vi "GetTypeDefs.vi"(0 "ClassReaderNative in":refnum<class "ClassReaderNative.lvclass">, 5 "error in (no error)":errorcluster) -> (14 "ClassReaderNative out":refnum<class "ClassReaderNative.lvclass">, 15 "TypeDefs":T1[](array[typedef]), 19 "error out":errorcluster)   [LabVIEW 2012, in "ClassReaderNative.lvclass"]
uses:
  <resource>/Framework/Providers/Open_GDS/ClassProviders/Provider_LvNativeClass/ClassReaderNative_class/ClassReaderNative.lvclass
  <resource>/Framework/Providers/Open_GDS/UML/ReversedEngineering/ReversedEngineering TypeDefType.ctl
  <resource>/Framework/Providers/Open_GDS/UML/ReversedEngineering/ReversedEngineering AttributeInfoType.ctl
  <resource>/Framework/Providers/Open_GDS/ClassProviders/Common/CommonVIs/CommonVIs_AttributeDataType.ctl
  <resource>/Framework/Providers/Open_GDS/UML/UMLEditor/UMLEditor_VisibilityType.ctl
  <resource>/Framework/Providers/Open_GDS/ClassProviders/Provider_LvNativeClass/ClassReaderNative_class/ClassReaderNative.lvclass/ClassReaderNative.ctl
  <resource>/Framework/Providers/Open_GDS/ClassProviders/Provider_BaseClassInterface/ClassReader_class/ClassReader.lvclass
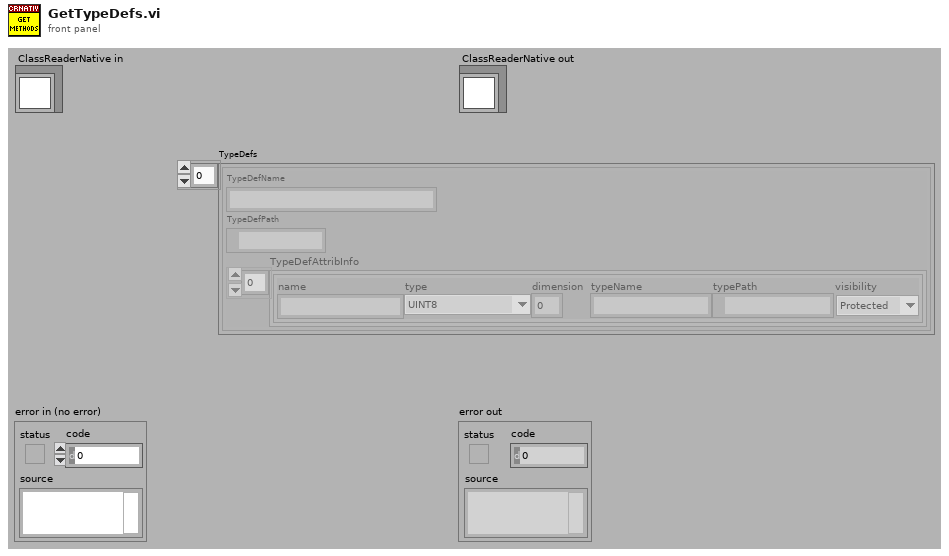
[diagram p1: front panel]
types:
  T1 = typedef "ReversedEngineering TypeDefType.ctl" = cluster{"TypeDefName":string, "TypeDefPath":path, "TypeDefAttribInfo":T2[]}
  T2 = typedef "ReversedEngineering AttributeInfoType.ctl" = cluster{"name":string, "type":T3, "dimension":i32, "typeName":string, "typePath":path, "visibility":T4}
  T3 = typedef "CommonVIs_AttributeDataType.ctl" = enum16{"UINT8", "INT8", "UINT16", "INT16", "UINT32", "INT32", "UINT64", "INT64", "SGL", "DBL", "EXT", "CSG", "CDB", "CXT", "TimeStamp", "STRING", "PATH", "BOOL", "ENUM", "RefNum", "VIRefNum", "LabVIEW Class", "Cluster", "Variant", "TypeDef", "Waveform", "LabVIEW Object", "Other"}
  T4 = typedef "UMLEditor_VisibilityType.ctl" = enum16{"Public", "Private", "Protected"}
  T5 = enum32{"invalid VI type", "Standard VI", "Control VI", "Global VI", "Polymorphic VI", "Configuration VI", "SubSystem", "Facade VI", "Method VI", "Statechart Diagram VI"}
  T6 = enum32{"not a control VI", "control", "typedef", "strict typedef"}
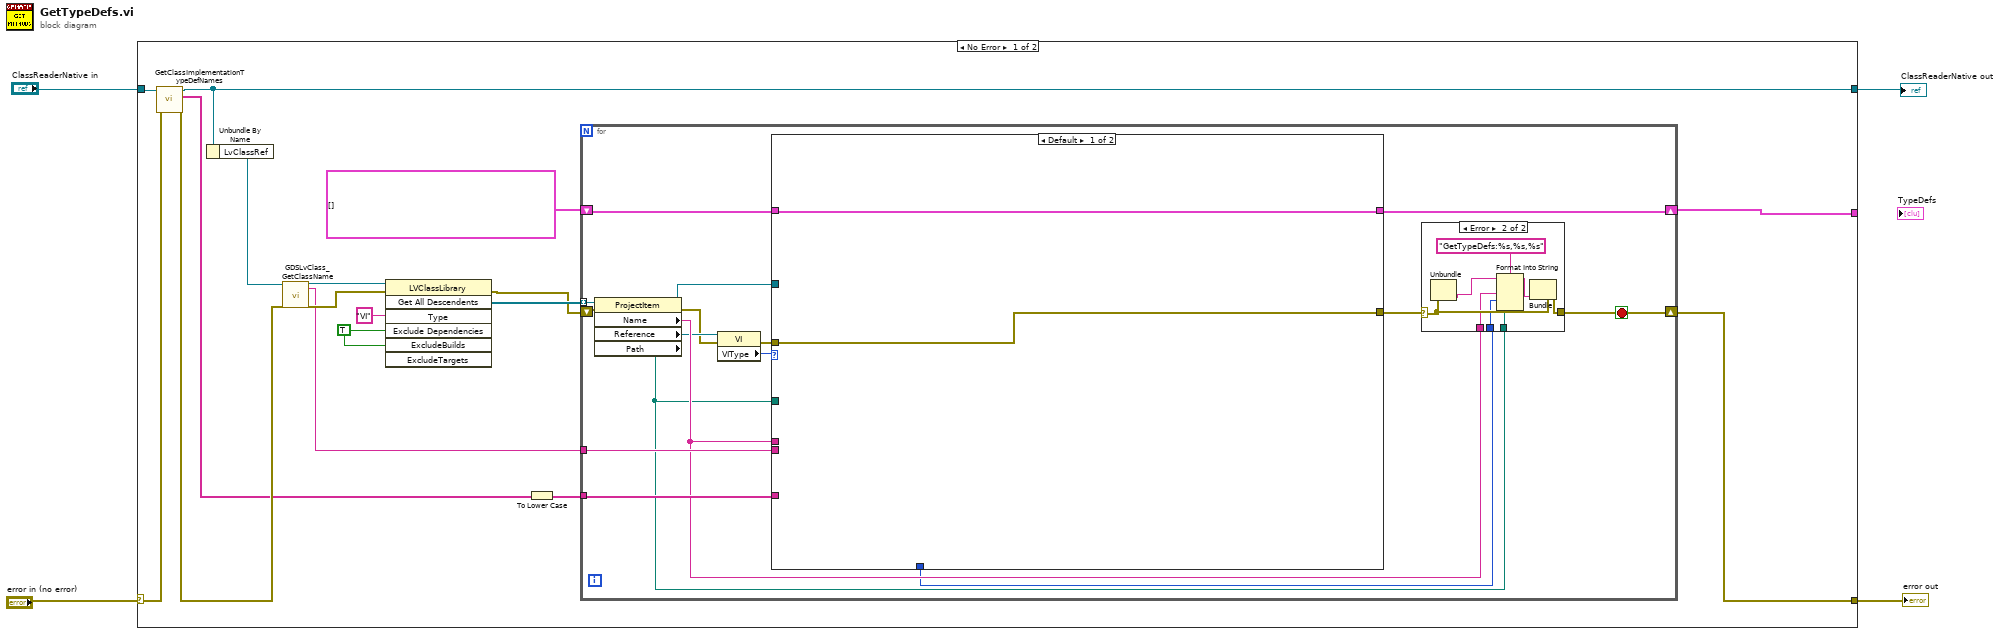
[diagram p0: block diagram]
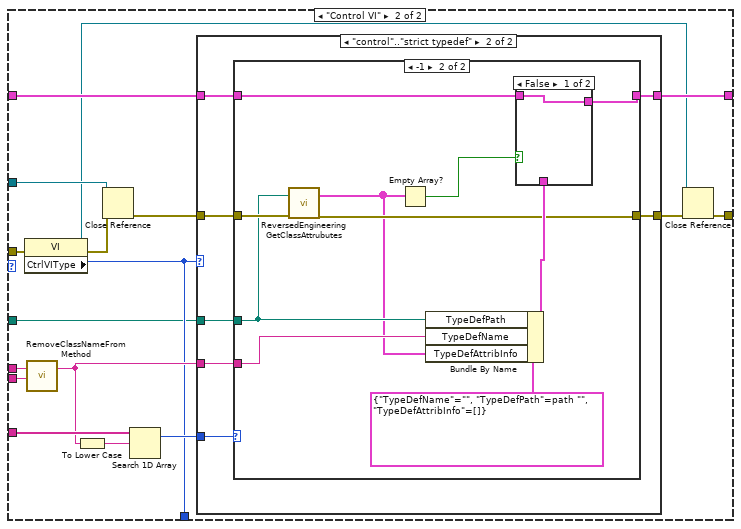
[diagram p2: hidden frame]
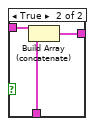
[diagram p5: hidden frame]
diagram:
  n1 = case shown="No Error" "error in (no error)" {
    selector: "error in (no error)" -> [w10 w91]
    tunnel: "ClassReaderNative in" -> [w11 w92]
    tunnel: [w8 w92] -> w2
    tunnel: [w14 _] -> _
    tunnel: [w6 w91] -> w1
    frame No Error {
      w5 = TRUE ("ExcludeDependencies")
      n2 = call-dynamic "GetClassImplementationTypeDefNames.vi"("error in (no error)"=w10, "ClassReaderNative in"=w11) -> ("error out"=w9:errorcluster, "ImplementationMethodNames"=w7:string[], "ClassReaderNative out"=w8:refnum<class "ClassReaderNative.lvclass">)  [unwired: 7 in]
      n3 = Unbundle By Name(w8) -> ("LvClassRef"=w15:refnum<vi>)
      n4 = call <resource>:"GDSLvClass_GetClassName.vi"("ViRef/Path,LvClassRef/Path"=w15, "error in (no error)"=w9) -> ("ClassRef"=w18:refnum<vi>, "ClassName(without .lvclass)"=w16:string, "error out"=w17:errorcluster)  [unwired: 15 in]
      n5 = invoke class="LVClassLibrary" method="Get All Descendents"(reference=w18, error in=w17, "Type"="VI", "Exclude Dependencies"=w5, "ExcludeBuilds"=w5) -> (error out=w19:errorcluster, "All Descendents"=w20:refnum<vi>[])  [unwired: 2 in, 5 out]
      n6 = To Lower Case(string=w7) -> (all lower case string=w13:string[])
      n7 = for {
        tunnel: w20 -> [w37] mode=indexing
        shift-right: [w29] -> w6
        shift-left: w19 -> [w36]
        shift-right: [w34] -> w14
        shift-left: T1[] [] ("TypeDefs") -> [w35]
        tunnel: w16 -> [w32]
        tunnel: w13 -> [w31]
        stop <- w29 stop-if-true
        n8 = property class="ProjectItem"(reference=w37, error in=w36) -> (reference out=w33:refnum<vi>, error out=w24:errorcluster, "Name"=w28:string, "Reference"=w25:refnum<vi>, "Path"=w26:path)
        n9 = property class="VI"(reference=w25, error in=w24) -> (error out=w23:errorcluster, "VIType"=w22:T5)  [unwired: 1 out]
        n10 = case shown="Default" w22 {
          tunnel: w35 -> [w39 w56]
          tunnel: [w39 w55] -> w34
          tunnel: w33 -> [_ w54]
          tunnel: w32 -> [_ w53]
          tunnel: w31 -> [_ w51]
          tunnel: [w38 w44] -> w30
          tunnel: w28 -> [_ w43]
          tunnel: [_ w42] -> w27
          tunnel: w26 -> [_ w41]
          tunnel: w23 -> [w38 w40]
          frame Default {
          }
          frame "Control VI" {
            n11 = property class="VI"(error in=w40) -> (reference out=w45:refnum<vi>, error out=w49:errorcluster, "CtrlVIType"=w42:T6)  [unwired: 1 in]
            n12 = call <resource>:"RemoveClassNameFromMethod.vi"("MethodVINameIn"=w43, "ClassName"=w53) -> ("MethodVINameOut"=w48:string)  [unwired: 17 in]
            n13 = To Lower Case(string=w48) -> (all lower case string=w50:string)
            n14 = Close Reference(reference=w54, error in (no error)=w49) -> (error out=w47:errorcluster)
            n15 = Search 1D Array(1D array=w51, element=w50) -> (index of element=w52:i32)  [unwired: 1 in]
            n16 = case shown="\"control\"..\"strict typedef\"" w42 {
              tunnel: w56 -> [w58 w65]
              tunnel: [w58 w64] -> w55
              tunnel: w52 -> [_ w63]
              tunnel: w41 -> [_ w62]
              tunnel: w48 -> [_ w61]
              tunnel: w47 -> [w57 w60]
              tunnel: [w57 w59] -> w46
              frame Default {
              }
              frame "control".."strict typedef" {
                n17 = case shown="-1" w63 {
                  tunnel: w65 -> [w67 w77]
                  tunnel: [w67 w76] -> w64
                  tunnel: w62 -> [_ w71]
                  tunnel: w61 -> [_ w73]
                  tunnel: w60 -> [w66 w72]
                  tunnel: [w66 w70] -> w59
                  frame 0, Default {
                  }
                  frame -1 {
                    n18 = call <resource>:"ReversedEngineering GetClassAttrubutes.vi"("Path(CtrlRenumf used if Path is empty)"=w71, "error in (no error)"=w72) -> ("attributeInfo"=w69:T2[], "error out"=w70:errorcluster)  [unwired: 15 in, 1 out]
                    n19 = Empty Array?(array=w69) -> (empty?=w68:bool)
                    n20 = Bundle By Name(cluster=T1 {"TypeDefName"="", "TypeDefPath"=path "", "TypeDefAttribInfo"=[]} ("TypeDef"), "TypeDefPath"=w71, "TypeDefName"=w73, "TypeDefAttribInfo"=w69) -> (w74:T1)
                    n21 = case shown="False" w68 {
                      tunnel: w77 -> [w78 w81]
                      tunnel: [w78 w80] -> w76
                      tunnel: w74 -> [_ w79]
                      frame False {
                      }
                      frame True {
                        n22 = Build Array (concatenate)(w81, w79) -> (w80:T1[])
                      }
                    }
                  }
                }
              }
            }
            n23 = Close Reference(reference=w45, error in (no error)=w46) -> (error out=w44:errorcluster)
          }
        }
        n24 = case shown="Error" w30 {
          selector: w30 -> [w82 w90]
          tunnel: [w82 w89] -> w29
          tunnel: w28 -> [_ w85]
          tunnel: w27 -> [_ w84]
          tunnel: w26 -> [_ w83]
          frame No Error {
          }
          frame Error {
            n25 = Unbundle(w90) -> ("source"=w88:string)  [unwired: 2 out]
            n26 = Format Into String(format string="GetTypeDefs:%s,%s,%s", initial string=w88, w85, w84, w83) -> (resulting string=w87:string)  [unwired: 1 in, 1 out]
            n27 = Bundle(cluster=w90, "source"=w87) -> (w89:errorcluster)  [unwired: 2 in]
          }
        }
      }
    }
    frame Error {
    }
  }
  "ClassReaderNative out" <- w2
  "error out" <- w1
